vi "PPAS_AUTOCMD_CMD_AUTO_SWERVE.vi"(6 "Pass_Through_Time":dbl=-1.0 format="%33.4f", 8 "Init":bool) -> (0 "AtReference":bool, 1 "Complete":bool, 3 "Chassis Velocity Target SI":T1 {"vOmega" format="%10.3f"; "vY" format="%10.3f"; "vX" format="%10.3f"})   [LabVIEW 2019]
uses:
  <vilib>/Rock Robotics/WPI/ThirdParty/JAS_Junk/TrajLib/Trajectory_Library.lvlib
  PPAS_AUTOCMD_GLOBALS.vi
  <vilib>/Rock Robotics/WPI/ThirdParty/MJansen/PathPlanner/PathPlanner24.lvlib
  <vilib>/Rock Robotics/WPI/ThirdParty/JAS_Junk/TrajLib/TypeDef/CHASSIS_SPEEDS.ctl
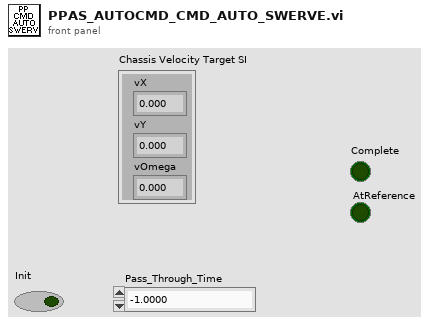
[diagram p1: front panel]
types:
  T1 = typedef "Trajectory_Library.lvlib/CHASSIS_SPEEDS.ctl" = cluster{"vX":dbl, "vY":dbl, "vOmega":dbl}
  T2 = typedef "PathPlanner24.lvlib/PathPlannerCmdPathPlannerAutoConfig.ctl" = cluster{"Command":T3, "ChoreoAuto":bool, "Version":string, "ResetOdom":bool, "Paths":T5[]}
  T3 = typedef "PathPlanner24.lvlib/PathPlannerCommandUtil.ctl" = cluster{"waitTime":dbl, "name":string, "pathName":string, "commands":cluster{"type":T4, "waitTime":dbl, "name":string, "pathName":string}[], "type":T4}
  T4 = typedef "PathPlanner24.lvlib/PathPlanner_CommandUtilType_ENUM.ctl" = enum16{"Unknown", "Wait", "Named", "Path", "Sequential", "Parallel", "Race", "Deadline"}
  T5 = typedef "PathPlanner24.lvlib/PathPlannerPath.ctl" = cluster{"Reversed":bool, "RotationTargets":T6[], "ConstraintZones":T8[], "EventMarkers":T10[], "GlobalConstraints":T9, "GoalEndState":T11, "AllPoints":T12[], "Name":string, "Waypoints":T14[], "PointTowardsZones":T15[], "IdealStartingState":T16, "IsChoreoPath":bool, "PreventFlipping":bool}
  T6 = typedef "PathPlanner24.lvlib/PathPlannerRotationTarget.ctl" = cluster{"position":dbl, "rotation":T7, "Exists":bool}
  T7 = typedef "Trajectory_Library.lvlib/ROTATION2D.ctl" = cluster{"VALUE":dbl, "COS":dbl, "SIN":dbl}
  T8 = typedef "PathPlanner24.lvlib/PathPlannerConstraintsZone.ctl" = cluster{"minPosition":dbl, "maxPosition":dbl, "Constraints":T9, "Present":bool}
  T9 = typedef "PathPlanner24.lvlib/PathPlannerPathConstraints.ctl" = cluster{"MaxVelocityMps;":dbl, "MaxAccelerationMpsSq;":dbl, "MaxAngularVelRadPsEc;":dbl, "MaxAngularAccRadPSecSq":dbl, "Exists":bool, "Unlimited":bool, "NominalVoltageVolts":dbl}
  T10 = typedef "PathPlanner24.lvlib/PathPlannerEventMarker.ctl" = cluster{"Position":dbl, "Command":T3, "TriggerName":string, "EndPosition":dbl}
  T11 = typedef "PathPlanner24.lvlib/PathPlannerGoalEndState.ctl" = cluster{"VelocityMPS":dbl, "Rotation":T7}
  T12 = typedef "PathPlanner24.lvlib/PathPlannerPathPoint.ctl" = cluster{"Position":T13, "DistAlongPath":dbl, "MaxV":dbl, "Constraints":T9, "RotationTarget":T6, "WaypointRelativePos":dbl}
  T13 = typedef "Trajectory_Library.lvlib/TRANSLATION2D.ctl" = cluster{"X":dbl, "Y":dbl}
  T14 = typedef "PathPlanner24.lvlib/PathPlannerWaypoint.ctl" = cluster{"prevControl":T13, "anchor":T13, "nextControl":T13, "PrevExists":bool, "NextExists":bool}
  T15 = typedef "PathPlanner24.lvlib/PathPlannerPointTowardsZone.ctl" = cluster{"RotationOffset":T7, "Name":string, "TargetPosition":T13, "MinPosition":dbl, "MaxPosition":dbl}
  T16 = typedef "PathPlanner24.lvlib/PathPlannerIdealStartingState.ctl" = cluster{"VelocityMPS":dbl, "Rotation":T7}
  T17 = typedef "Trajectory_Library.lvlib/PID_TUNING.ctl" = cluster{"Kp":dbl, "Ki":dbl, "Kd":dbl, "MaximumIntegral":dbl, "MinimumIntegral":dbl, "IntegralZone":dbl}
  T18 = typedef "Trajectory_Library.lvlib/POSE2D.ctl" = cluster{"TRANSLATION":T13, "ROTATION":T7}
  T19 = typedef "Trajectory_Library.lvlib/PROFILED_PID_CONTROLLER.ctl" = cluster{"Controller":T20, "Goal":T21, "Setpoint":T21, "Constraint":T22}
  T20 = typedef "Trajectory_Library.lvlib/PID_CONTROLLER.ctl" = cluster{"Kp":dbl, "Ki":dbl, "Kd":dbl, "Period":dbl, "Max_Integral":dbl, "Min_Integral":dbl, "Max_Input":dbl, "Min_Input":dbl, "Continuous":bool, "PositionError":dbl, "VelocityError":dbl, "PrevError":dbl, "Total_Integral":dbl, "PositionTolerance":dbl, "VelocityTolerance":dbl, "SetPoint":dbl, "Kf":dbl, "Prev_Deriv":dbl, "Prev_Deriv 2":dbl, "DerivativeFilter":bool, "Min_Output":dbl, "Max_Output":dbl, "Prev_F_P":dbl, "Prev_F_P_2":dbl, "AntiWindupActive":bool, "Measurement":dbl, "IntegralZone":dbl}
  T21 = typedef "Trajectory_Library.lvlib/TRAPEZOID_PROFILE_STATE.ctl" = cluster{"Position":dbl, "Velocity":dbl}
  T22 = typedef "Trajectory_Library.lvlib/TRAPEZOID_PROFILE_CONSTRAINT.ctl" = cluster{"MaxVelocity":dbl, "MaxAcceleration":dbl}
  T23 = typedef "Trajectory_Library.lvlib/HOLONOMIC_PACK_TUNING.ctl" = cluster{"X PID Tuning":T17, "Y PID Tuning":T17, "thetaProfiledPID_CTRL":T19}
  T24 = typedef "PathPlanner24.lvlib/PathPlannerCmdFollowHolConfig.ctl" = cluster{"HOLONOMIC_CTRL_PACK_TUNING":T23, "Max Wheel Speed M/S":dbl, "Tolerance SI":T18, "Drive Base Radius M":dbl, "ControlPastEnd_Sec":dbl, "Period_Sec":dbl, "Trigger Events":bool}
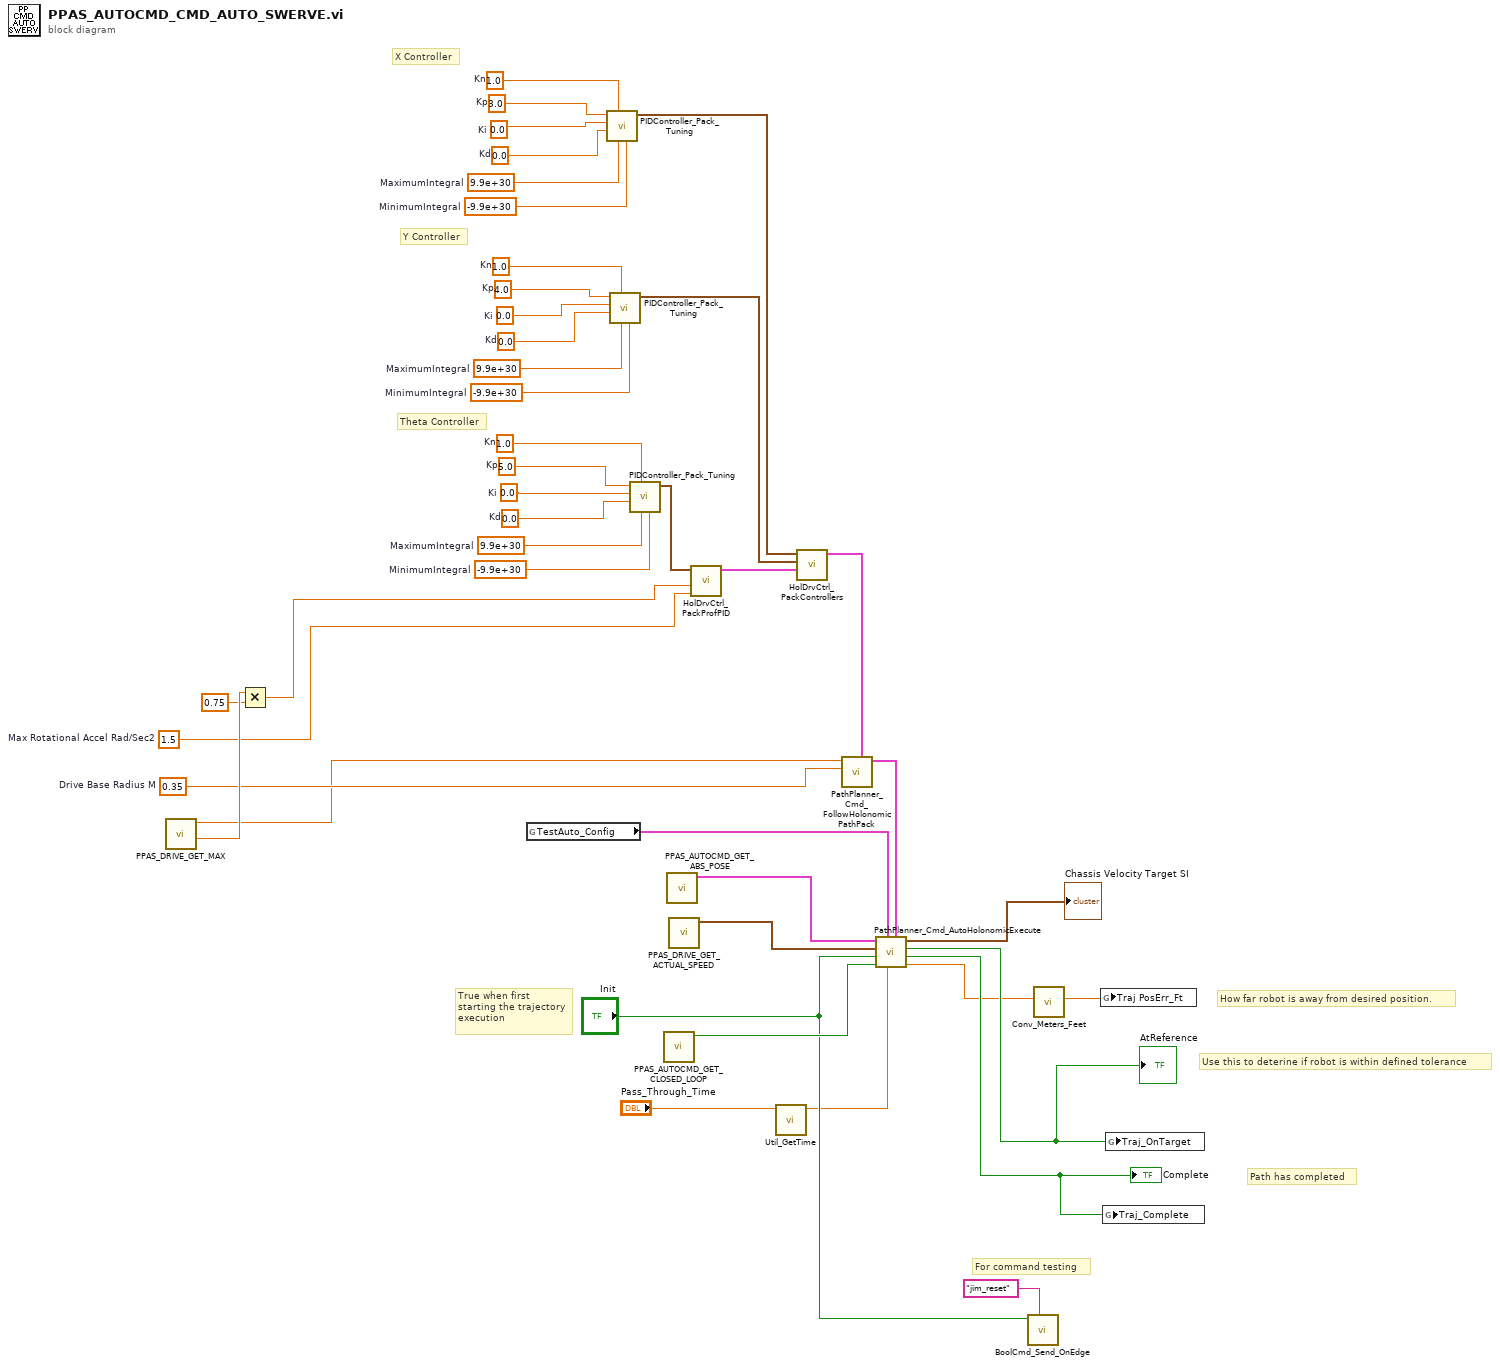
[diagram p0: block diagram]
diagram:
  w33 = 1.0  # Kn
  w30 = 5.0  # Kp
  w21 = 0.0  # Ki
  w20 = 0.0  # Kd
  w19 = 9.9e+30  # MaximumIntegral
  w18 = -9.9e+30  # MinimumIntegral
  w35 = 1.0  # Kn
  w32 = 3.0  # Kp
  w29 = 0.0  # Ki
  w28 = 0.0  # Kd
  w27 = 9.9e+30  # MaximumIntegral
  w26 = -9.9e+30  # MinimumIntegral
  w34 = 1.0  # Kn
  w31 = 4.0  # Kp
  w25 = 0.0  # Ki
  w24 = 0.0  # Kd
  w23 = 9.9e+30  # MaximumIntegral
  w22 = -9.9e+30  # MinimumIntegral
  w15 = 0.35  # Drive Base Radius M
  w16 = 1.5  # Max Rotational Accel Rad/Sec2
  # "For command testing"
  # "Path has completed"
  # "How far robot is away from desired position."
  # "Use this to deterine if robot is within defined tolerance"
  # "Theta Controller"
  # "Y Controller"
  # "X Controller"
  # "True when first\nstarting the trajectory\nexecution"
  n1 = call "PPAS_DRIVE_GET_MAX.vi"() -> ("Max Rotational Vel (Rad/Sec)"=w43:dbl, "Max Wheel Vel (Meter/Sec)"=w9:dbl)  [unwired: 10 in]
  n2 = Multiply(x=w43, y=0.75) -> (x*y=w17:dbl)
  n3 = global read "PPAS_AUTOCMD_GLOBALS.vi" "TestAuto_Config"() -> (w14:T2)
  n4 = call <vilib>:"PIDController_Pack_Tuning.vi"("MinimumIntegral"=w26, "MaximumIntegral"=w27, "Kn"=w35, "Kd"=w28, "Ki"=w29, "Kp"=w32) -> ("PID Tuning"=w39:T17)  [unwired: 5 in]
  n5 = call <vilib>:"PIDController_Pack_Tuning.vi"("MinimumIntegral"=w22, "MaximumIntegral"=w23, "Kn"=w34, "Kd"=w24, "Ki"=w25, "Kp"=w31) -> ("PID Tuning"=w40:T17)  [unwired: 5 in]
  n6 = call <vilib>:"PIDController_Pack_Tuning.vi"("MinimumIntegral"=w18, "MaximumIntegral"=w19, "Kn"=w33, "Kd"=w20, "Ki"=w21, "Kp"=w30) -> ("PID Tuning"=w36:T17)  [unwired: 5 in]
  n7 = call "PPAS_AUTOCMD_GET_CLOSED_LOOP.vi"() -> ("AUTO_CLOSED_LOOP"=w11:bool)  [unwired: 11 in]
  n8 = call "PPAS_AUTOCMD_GET_ABS_POSE.vi"() -> ("Absolute Odometry Pose"=w13:T18)  [unwired: 11 in]
  n9 = call "PPAS_DRIVE_GET_ACTUAL_SPEED.vi"() -> ("Drv Chassis Actual Velocity"=w12:T1)  [unwired: 11 in]
  n10 = call <vilib>:"HolDrvCtrl_PackProfPID.vi"("Max Accel"=w16, "Max Speed"=w17, "Theta PID Tuning"=w36) -> ("Theta PID CONTROLLER"=w41:T19)  [unwired: 8 in]
  n11 = call <vilib>:"Util_GetTime.vi"("Pass_Through_Time"="Pass_Through_Time") -> ("FPGA_Time_Seconds"=w1:dbl)  [unwired: 8 in, 2 out]
  n12 = call <vilib>:"HolDrvCtrl_PackControllers.vi"("thetaProfiledPID_CTRL"=w41, "Y PID Tuning"=w40, "X PID Tuning"=w39) -> ("HOLONOMIC_CTRL_PACK_TUNING"=w38:T23)  [unwired: 8 in]
  n13 = call <vilib>:"PathPlanner_Cmd_FollowHolonomicPathPack.vi"("HOLONOMIC_CTRL_PACK_TUNING"=w38, "Drive Base Radius M"=w15, "Max Wheel Speed M/S"=w9) -> ("PathPlanner_Ctrl_HolDrvConfig"=w37:T24)  [unwired: 8 in]
  n14 = call <vilib>:"PathPlanner_Cmd_AutoHolonomicExecute.vi"("PathPlanner_Cmd_FollowHolConfig"=w37, "PassthroughTime_SEC"=w1, "PathPlanner_Cmd_AutoConfig"=w14, "Enabled"=w11, "Reset"="Init", "CurrentChassisSpeeds"=w12, "Current Pose SI"=w13) -> ("Position Error M"=w4:dbl, "Complete"=w6:bool, "At Reference"=w7:bool, "calcChassisSpeed"=→"Chassis Velocity Target SI":T1)  [unwired: 1 in]
  "AtReference" <- w7
  "Complete" <- w6
  n15 = call <vilib>:"BoolCmd_Send_OnEdge.vi"("Command Name"="jim_reset", "Value"="Init") -> ()  [unwired: 9 in, 1 out]
  n16 = call <vilib>:"Conv_Meters_Feet.vi"("Meters"=w4) -> ("Feet"=w5:dbl)  [unwired: 10 in]
  n17 = global write "PPAS_AUTOCMD_GLOBALS.vi" "Traj PosErr_Ft"(w5) -> ()
  n18 = global write "PPAS_AUTOCMD_GLOBALS.vi" "Traj_Complete"(w6) -> ()
  n19 = global write "PPAS_AUTOCMD_GLOBALS.vi" "Traj_OnTarget"(w7) -> ()
